vi "SmartSEM Remote API FIB mode.vi"(5 "Wait (ms)":u32, 7 "Iterations":u32=3, 8 "error in":errorcluster, 10 "FIB mode":T1(ring), 11 "Api":refnum<k7>(container)) -> (0 "error out":errorcluster, 3 "Api out":refnum<k7>)   [LabVIEW 2018]
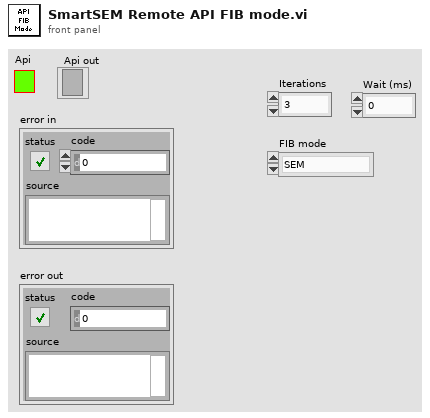
[diagram p1: front panel]
types:
  T1 = enum16{"SEM", "FIB", "Mill", "SEM + FIB", "Mill + SEM", "Drift SEM", "Drift FIB", "None", "Ext", "Ext + SEM"}
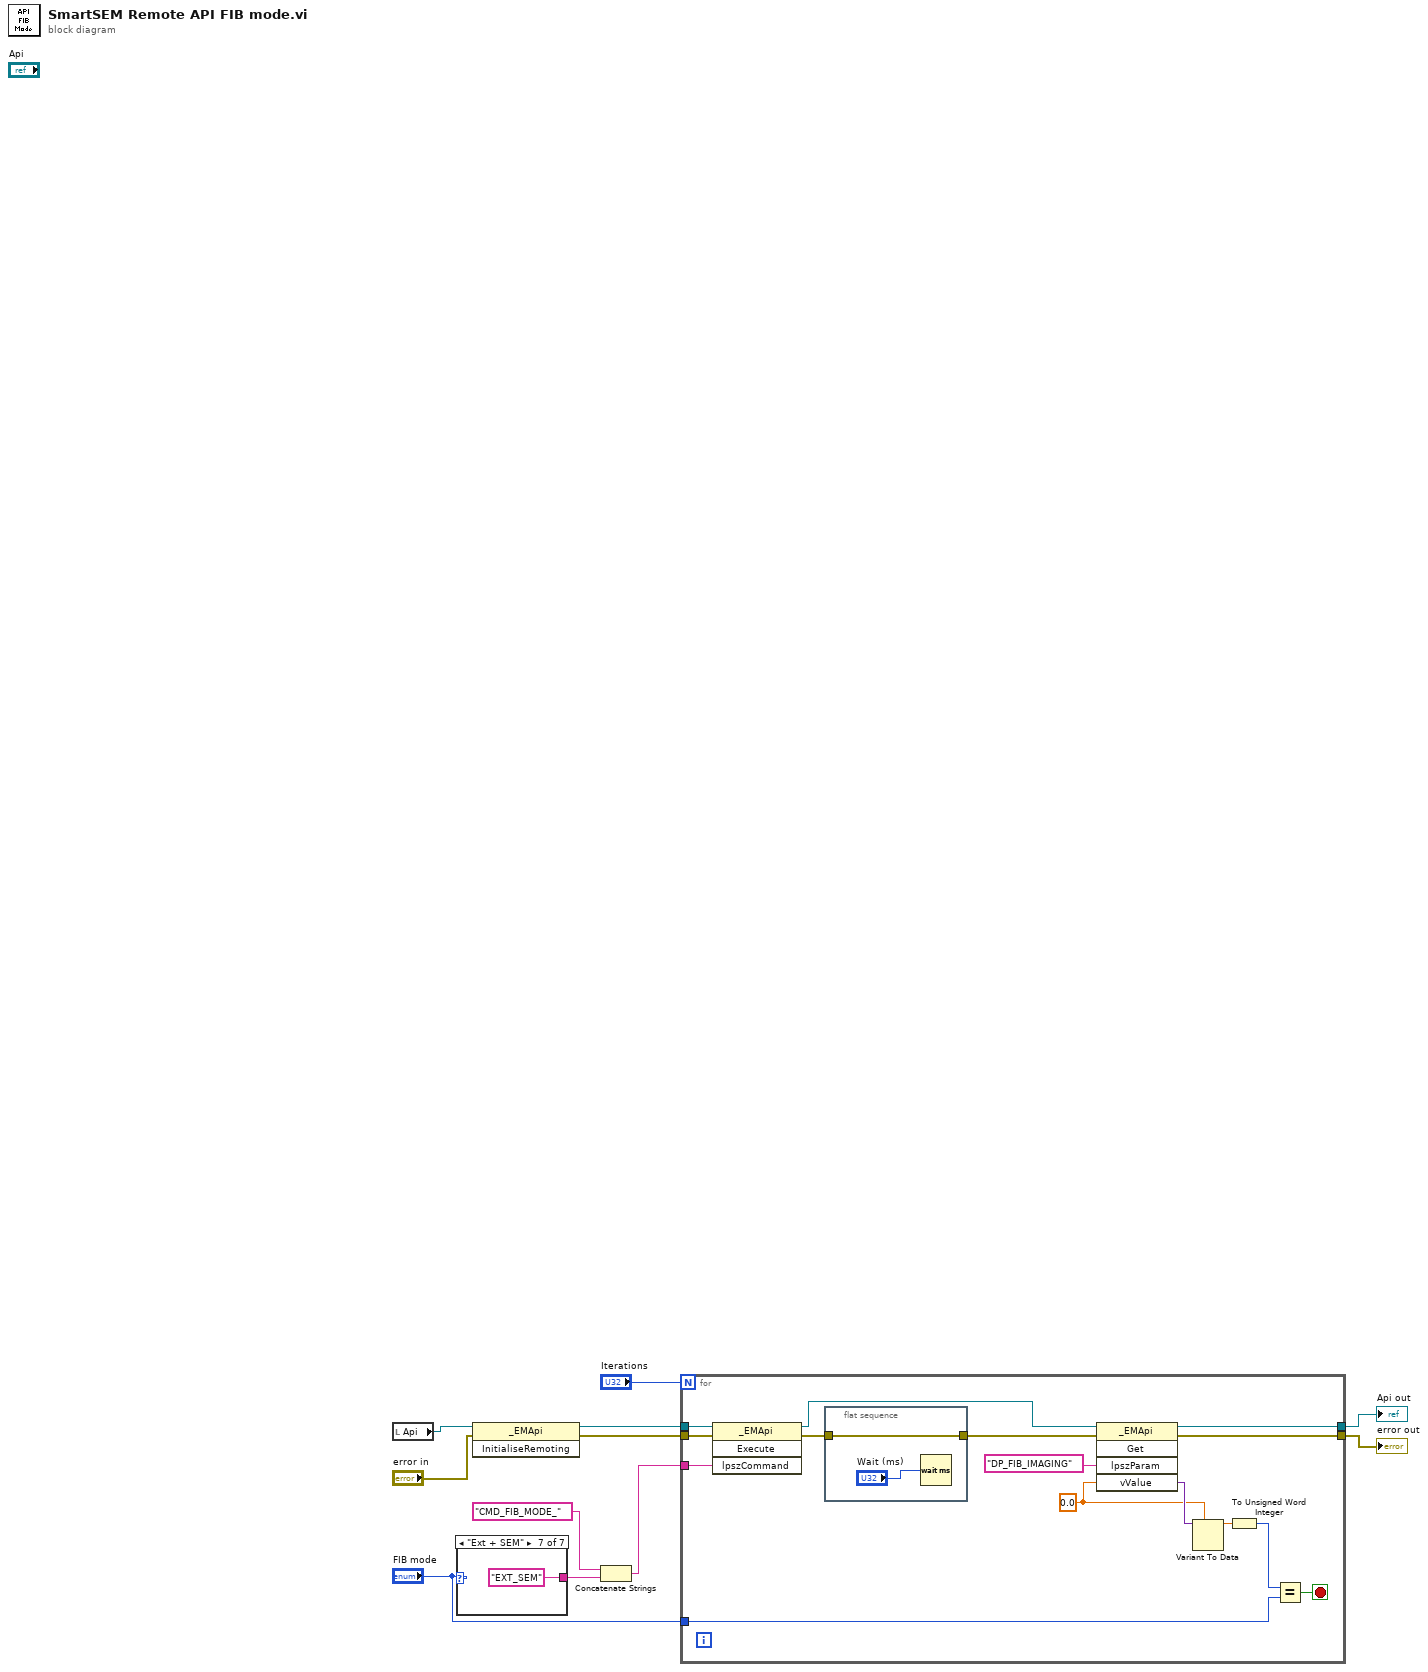
[diagram p0: block diagram]
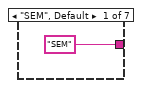
[diagram p2: hidden frame]
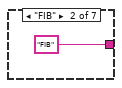
[diagram p3: hidden frame]
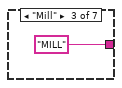
[diagram p4: hidden frame]
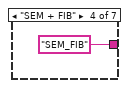
[diagram p5: hidden frame]
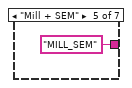
[diagram p6: hidden frame]
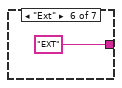
[diagram p7: hidden frame]
diagram:
  n1 = local read "Api"() -> (w11:refnum<k7>)
  n2 = case shown="\"Ext + SEM\"" "FIB mode" {
    tunnel: ["SEM" ("lpszCommand") "FIB" ("lpszCommand") "MILL" ("lpszCommand") "SEM_FIB" ("lpszCommand") "MILL_SEM" ("lpszCommand") "EXT" ("lpszCommand") "EXT_SEM" ("lpszCommand")] -> w8
    frame "SEM", Default {
    }
    frame "FIB" {
    }
    frame "Mill" {
    }
    frame "SEM + FIB" {
    }
    frame "Mill + SEM" {
    }
    frame "Ext" {
    }
    frame "Ext + SEM" {
    }
  }
  n3 = invoke class="_EMApi" method="InitialiseRemoting"(reference=w11, error in="error in") -> (reference out=w10:refnum<k7>, error out=w5:errorcluster)  [unwired: 1 in, 1 out]
  n4 = Concatenate Strings("CMD_FIB_MODE_" ("lpszCommand"), w8) -> (w7:string)
  n5 = for {
    N: "Iterations" -> [_]
    tunnel: w10 -> [w33]
    tunnel: w7 -> [w32]
    tunnel: "FIB mode" -> [w25]
    tunnel: w5 -> [w23]
    tunnel: [w22] -> w3
    tunnel: [w21] -> w4
    stop <- w24 stop-if-true
    w28 = sgl 0.0
    n6 = invoke class="_EMApi" method="Execute"(reference=w33, error in=w23, "lpszCommand"=w32) -> (reference out=w31:refnum<k7>, error out=w20:errorcluster)  [unwired: 1 in, 2 out]
    n7 = flat-sequence {
      tunnel: [w35] -> w19
      tunnel: w20 -> [w35]
      frame #0 {
        n8 = Wait (ms)(milliseconds to wait="Wait (ms)") -> ()  [unwired: 1 out]
      }
    }
    n9 = invoke class="_EMApi" method="Get"(reference=w31, error in=w19, "lpszParam"="DP_FIB_IMAGING", "vValue"=w28) -> (reference out=w22:refnum<k7>, error out=w21:errorcluster, "vValue"=w29:variant)  [unwired: 1 in, 2 out]
    n10 = Variant To Data(type=w28, Variant=w29) -> (data=w27:sgl)  [unwired: 1 in, 1 out]
    n11 = To Unsigned Word Integer(number=w27) -> (unsigned 16bit integer=w26:u16)
    n12 = Equal?(x=w26, y=w25) -> (x = y?=w24:bool)
  }
  "Api out" <- w3
  "error out" <- w4
